vi "AB Tutorial Analyze.vi"(9 "WFChart Refnum":refnum<vi>, 10 "Datafile path":path, 11 "Array In":dbl[](array[numeric])) -> (1 "Array Out":dbl[][](array[numeric]))   [LabVIEW 2019]
doc: "This VI is part of an example program for how to use the Application Builder. For more information about this example program please refer to the top level VI \"AB Tutorial GUI.vi\" or the LabVIEW Help for Application Builder."
uses:
  <vilib>/Utility/file.llb/Read From Spreadsheet File (DBL).vi
panel:
  # "rearrange this so that Array Out and Array In are in same location"
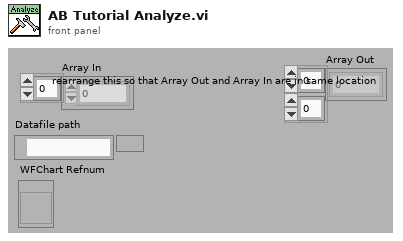
[diagram p1: front panel]
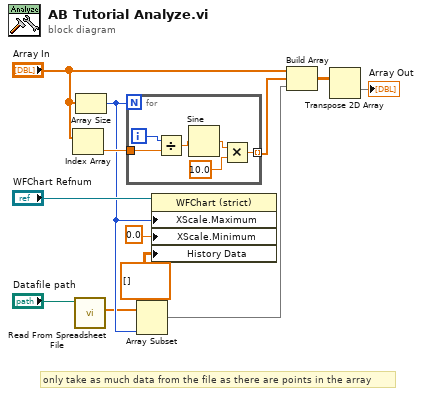
[diagram p0: block diagram]
diagram:
  # "only take as much data from the file as there are points in the array"
  n1 = Index Array(array="Array In") -> (element=w10:dbl)  [unwired: 1 in]
  n2 = call-poly <vilib>:"Read From Spreadsheet File.vi"("file path (dialog if empty)"="Datafile path") -> ("first row"=w2:dbl[])  [unwired: 6 in, 4 out]
  n3 = Array Size(array="Array In") -> (size(s)=w6:i32)
  n4 = for {
    N: w6 -> [_]
    tunnel: [w15] -> w12 mode=indexing
    tunnel: w10 -> [w13]
    i -> [w14]
    n5 = Divide(x=w14, y=w13) -> (x/y=w18:dbl)
    n6 = Sine(x=w18) -> (sin(x)=w17:dbl)
    n7 = Multiply(x=w17, y=10.0) -> (x*y=w15:dbl)
  }
  n8 = Array Subset(array=w2, length=w6) -> (w5:dbl[])  [unwired: 1 in]
  n9 = property class="WFChart (strict)"(reference="WFChart Refnum", "XScale.Maximum"=w6, "XScale.Minimum"=0.0 ("y"), "History Data"=dbl[][] []) -> ()  [unwired: 1 in, 2 out]
  n10 = Build Array("Array In", w12, w5) -> (w3:dbl[][])
  n11 = Transpose 2D Array(2D array=w3) -> (transposed array=→"Array Out":dbl[][])
